vi "motor run nonloop.vi"(8 "Error In":errorcluster, 9 "Reset":bool, 10 "Speed (RPM)":dbl, 11 "Motor single.lvclass":refnum<class "Motor single.lvclass">) -> (0 "error out":errorcluster, 1 "setpoint":dbl, 2 "encoder out":i32, 3 "output cluster":refnum<class "Motor single.lvclass">, 4 "PID output":dbl format="%.2f")   [LabVIEW 2019, in "Motor single.lvclass"]
uses:
  Motor single.lvclass
  Motor single.lvclass/Motor single.ctl
  motor control & config.ctl
  <vilib>/addons/control/pid/pid.llb/PID (DBL).vi
  <vilib>/addons/control/pid/NI_PID_pid.lvlib
panel:
  out "Frequence":dbl
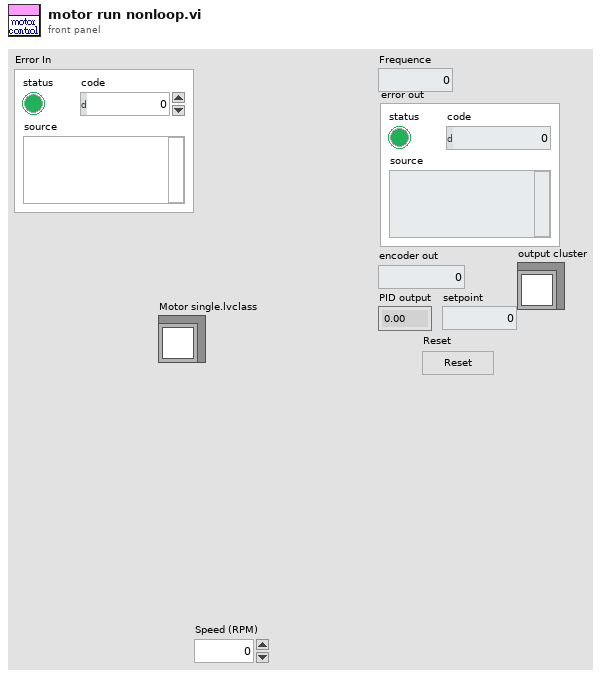
[diagram p1: front panel]
types:
  T1 = cluster{"proportional gain (Kc)":dbl, "integral time (Ti, min)":dbl, "derivative time (Td, min)":dbl}
  T2 = typedef "Motor single.lvclass/motor control & config.ctl" = enum16{"control", "config"}
  T3 = typedef "Motor single.lvclass/motor enum(FPGA).ctl" = enum16{"M1", "M2", "M3", "M4"}
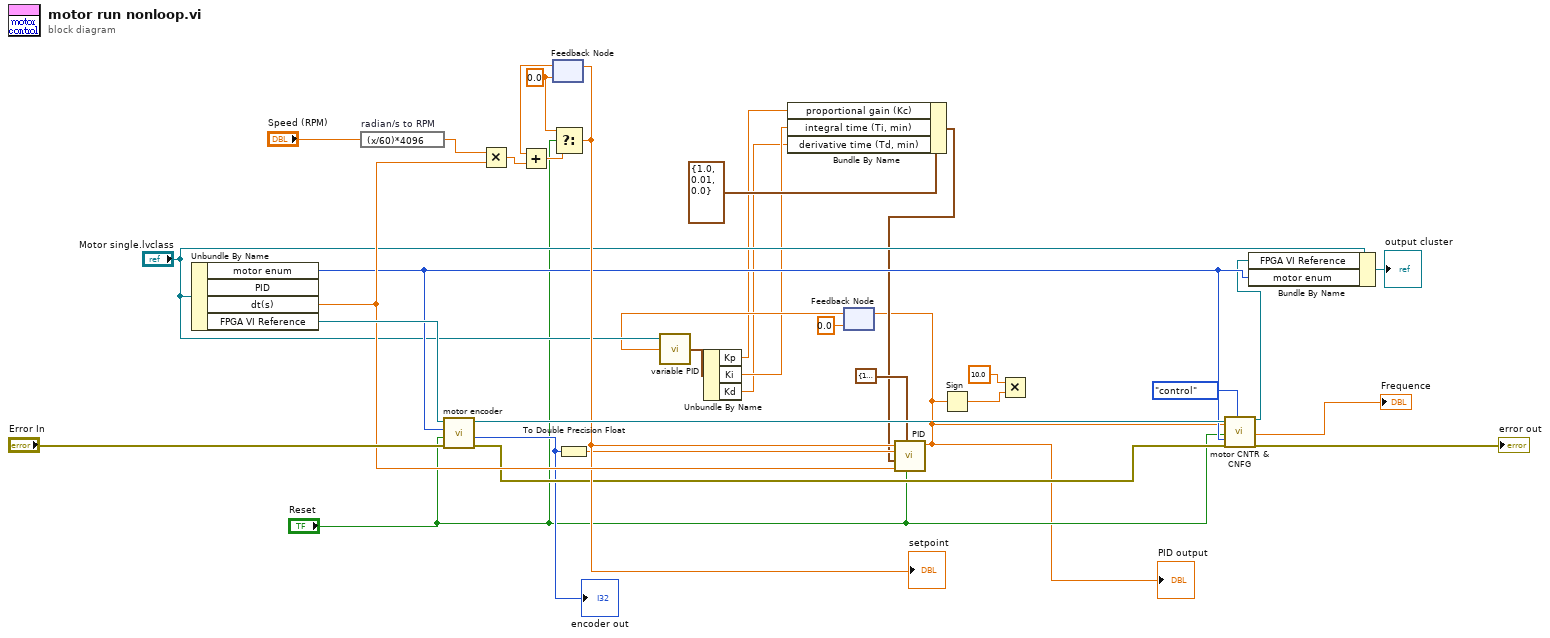
[diagram p0: block diagram]
diagram:
  w24 = 0.0
  n1 = Unbundle By Name("Motor single.lvclass") -> ("motor enum"=w18:T3, "dt(s)"=w28:dbl, "FPGA VI Reference"=w34:refnum<k20>)  [unwired: 1 out]
  n2 = expression code="(x/60)*4096" "radian/s to RPM"("Speed (RPM)") -> (w29:dbl)
  n3 = call "motor encoder.vi"("Error In"="Error In", "Motor Reset"="Reset", "Motor Enum"=w18, "FPGA VI Reference In"=w34) -> ("Error Out"=w22:errorcluster, "encoder out"=w20:i32, "FPGA VI Reference Out"=w33:refnum<k20>)  [unwired: 5 in]
  "encoder out" <- w20
  n4 = Multiply(x=w29, y=w28) -> (x*y=w25:dbl)
  n5 = feedback #1(w24) -> (w26:dbl)
  n6 = Add(x=w26, y=w25) -> (x+y=w27:dbl)
  n7 = Select(t=w24, s="Reset", f=w27) -> (s? t:f=w23:dbl)
  "setpoint" <- w23
  n8 = feedback-in #1(w23) -> ()
  n9 = To Double Precision Float(number=w20) -> (double precision float=w21:dbl)
  n10 = feedback #2(0.0 ("dt out (s)")) -> (w12:dbl)
  n11 = call "variable PID.vi"("PID output"=w12, "Motor single.lvclass"="Motor single.lvclass") -> ("PID"=w9:cluster{"Kp":dbl, "Ki":dbl, "Kd":dbl})  [unwired: 1 in]
  n12 = Unbundle By Name(w9) -> ("Kp"=w7:dbl, "Ki"=w6:dbl, "Kd"=w5:dbl)
  n13 = Bundle By Name(cluster=T1 {"proportional gain (Kc)"=1.0, "integral time (Ti, min)"=0.01, "derivative time (Td, min)"=0.0} ("PID gains"), "proportional gain (Kc)"=w7, "integral time (Ti, min)"=w6, "derivative time (Td, min)"=w5) -> (w4:T1)
  n14 = call-poly <vilib>:"PID.vi"("reinitialize? (F)"="Reset", "output range"=cluster{"output high":dbl, "output low":dbl} {"output high"=100.0, "output low"=-100.0}, "dt (s)"=w28, "PID gains"=w4, "process variable"=w21, "setpoint"=w23) -> ("output"=w1:dbl)  [unwired: 4 in, 1 out]
  "PID output" <- w1
  n15 = feedback-in #2(w1) -> ()
  n16 = Sign(1:w1) -> (0:w2:dbl)
  n17 = Multiply(x=10.0, y=w2) -> ()  [unwired: 1 out]
  n18 = call "motor CNTR & CNFG.vi"("FPGA VI Reference"=w33, "speed duty cycle"=w1, "Motor Brake"="Reset", "Motor select"=w18, "Error In"=w22, "Function"=motor_control_&_config."control") -> ("FPGA VI Reference Out"=w17:refnum<k20>, "Frequence"=→"Frequence":dbl, "error out"=→"error out":errorcluster)  [unwired: 11 in]
  n19 = Bundle By Name(cluster="Motor single.lvclass", "FPGA VI Reference"=w17, "motor enum"=w18) -> (→"output cluster":refnum<class "Motor single.lvclass">)
